vi "RelayControlPlottingSBE37andRTD.vi"() -> ()   [LabVIEW 2020]
uses:
  <vilib>/Utility/file.llb/Write Delimited Spreadsheet (string).vi
  <vilib>/Instr/_visa.llb/VISA Configure Serial Port (Instr).vi
  <vilib>/Utility/file.llb/Read Delimited Spreadsheet (string).vi
  75e3b035-2a18-8740-ad09-42cbc6dca646.vi
  3107c4ef-b790-5349-8479-afe5556ad064.vi
  <vilib>/picture/cartesn2.llb/XY Plot Type.ctl
panel:
  in  "setpoint":dbl format="%.2f"
  in  "XY plot cosmetics":T2={"plot color"=16776960, "XY plot type"=enum."connected points", "baseline"=0.0} {"baseline" format="%0.2f"}
  in  "cartesian axis attributes":T3={"x minimum"=0.0, "x maximum"=0.0, "x log?"=FALSE, "x precision"=1, "x format"=enum."Decimal", "y minimum"=0.0, "y maximum"=0.0, "y log?"=FALSE, "y precision"=1, "y format"=enum."Decimal"} {"x minimum" format="%0.2f"; "x maximum" format="%0.2f"; "y minimum" format="%0.2f"; "y maximum" format="%0.2f"}
  out "Table Control 2":string[][](table)
  out "2D Picture 3":picture
  out "Thermometer":dbl(slide) scale=0.0..100.0
  out "Table Control":string[][](table)
  out "2D Picture":picture
  out "Response":string
  out "?":u32
  in  "VISA resource name":refnum<visa-resource-name>="COM1"
  in  "error in (no error)":errorcluster
  in  "stop":bool
  in  "format (%s)":string="%s"
  out "error out":errorcluster
  in  "VISA resource name 2":refnum<visa-resource-name>
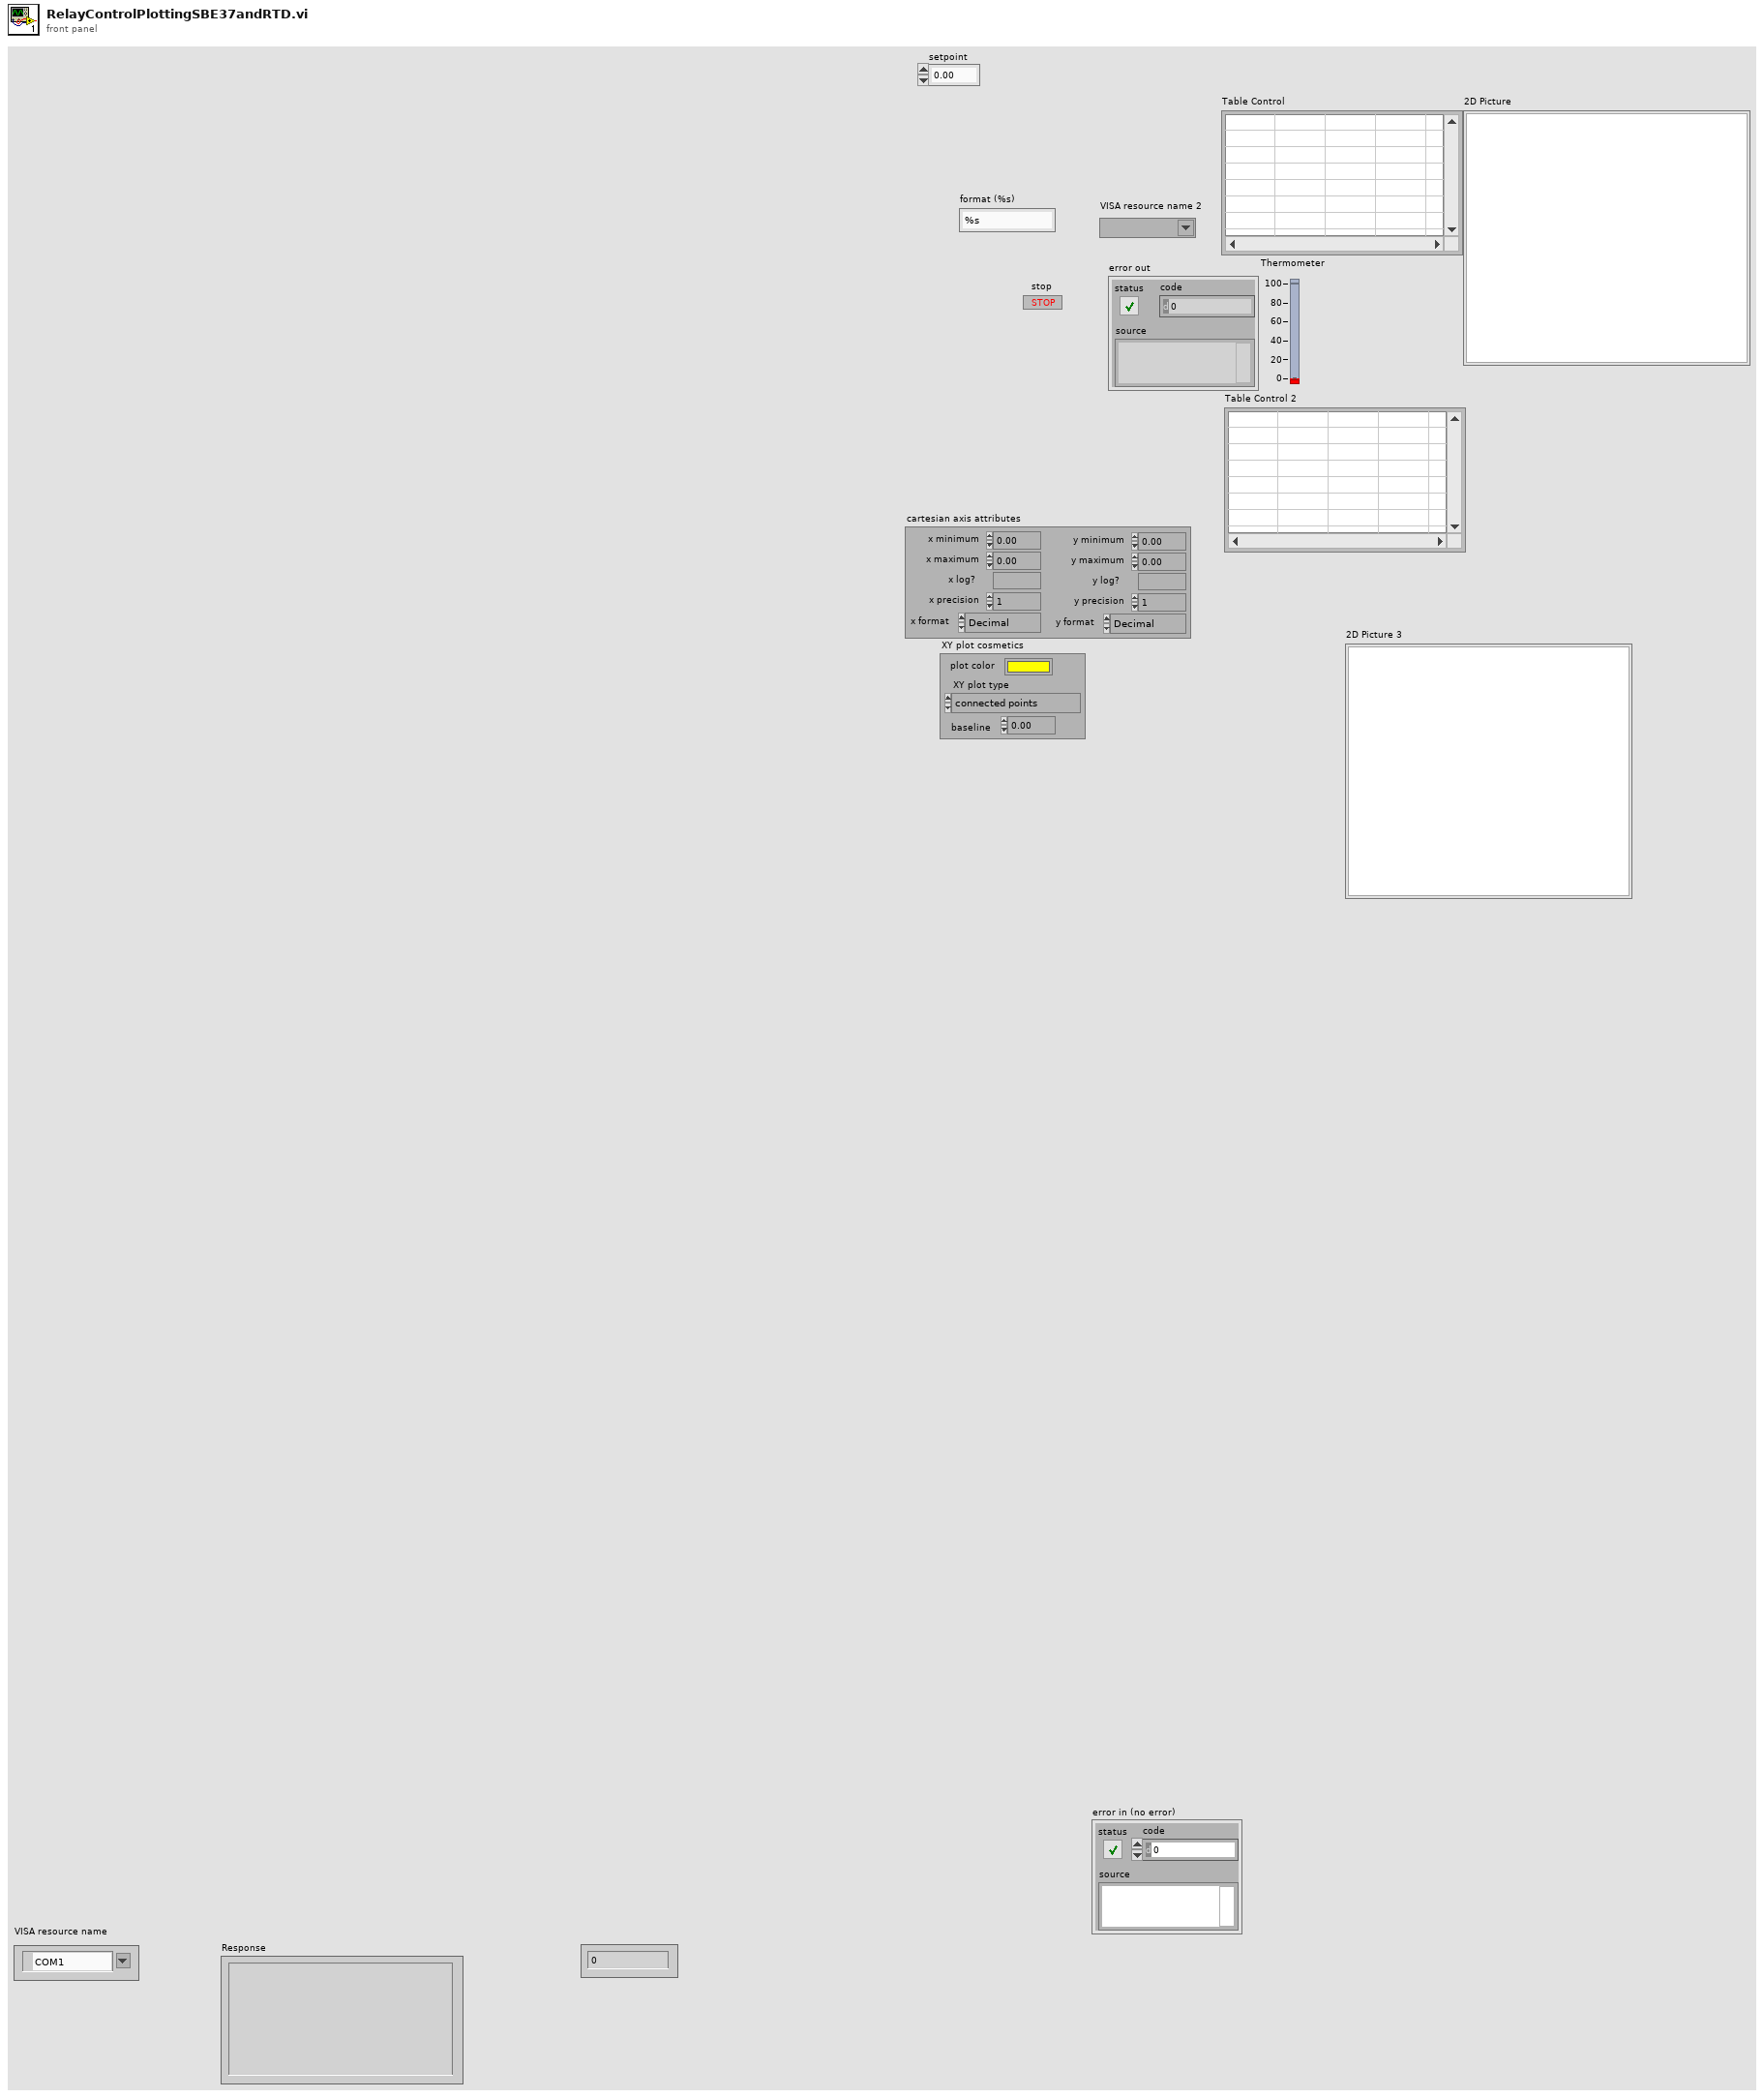
[diagram p1: front panel]
types:
  T1 = typedef "XY Plot Type.ctl" = enum16{"points", "squares", "circles", "connected points", "connected squares", "connected circles", "comb plot", "sized scatter plot", "sized-colored scatter plot", "min-max lines"}
  T2 = cluster{"plot color":u32, "XY plot type":T1, "baseline":dbl}
  T3 = cluster{"x minimum":dbl, "x maximum":dbl, "x log?":bool, "x precision":u8, "x format":enum8{"Decimal", "Scientific", "Engineering", "Binary", "Octal", "Hex"}, "y minimum":dbl, "y maximum":dbl, "y log?":bool, "y precision":u8, "y format":enum8{"Decimal", "Scientific", "Engineering", "Binary", "Octal", "Hex"}}
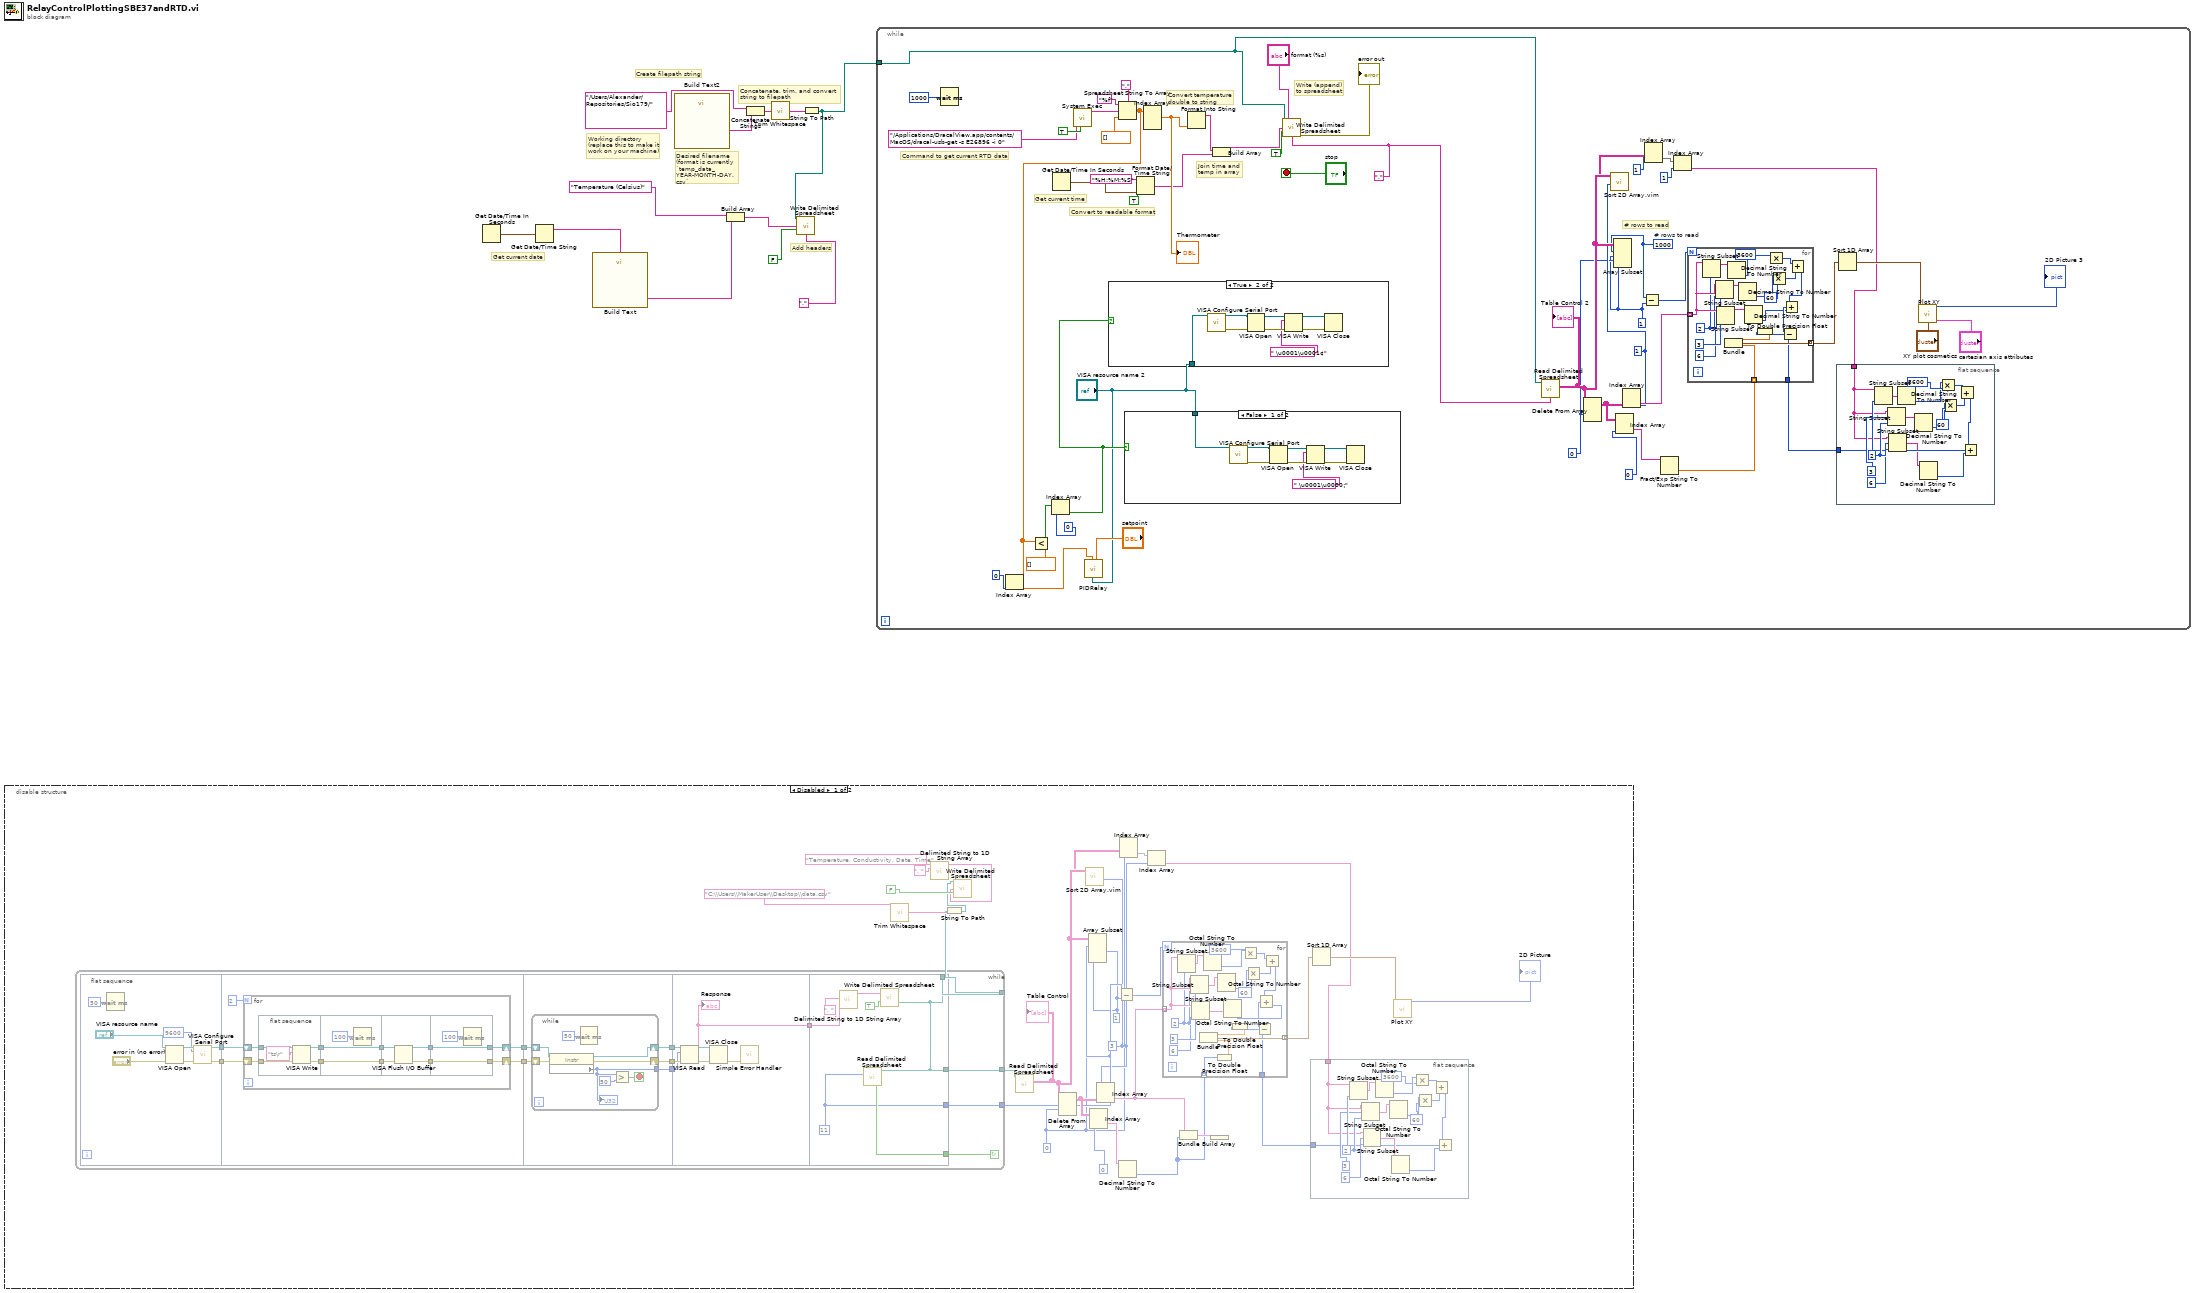
[diagram p0: block diagram]
diagram:
  # "Add headers"
  # "Get current date"
  # "Concatenate, trim, and convert string to filepath"
  # "Desired filename (format is currently `temp_data_YEAR-MONTH-DAY.csv`"
  # "Working directory (replace this to make it work on your machine)"
  # "Create filepath string"
  n1 = disable-structure shown="Disabled" {
    frame Disabled {
      w17 = 1
      w14 = 3
      w13 = 0
      n2 = call <vilib>:"Trim Whitespace.vi"("string"="C:\\Users\\MakerUser\\Desktop\\data.csv") -> ("trimmed string"=w38:string)  [unwired: 1 in]
      n3 = call <vilib>:"Delimited String to 1D String Array.vi"("delimiter"=", ", "delimited string"="Temperature, Conductivity, Date, Time") -> ("string array"=w35:string[])  [unwired: 9 in]
      n4 = String To Path(string=w38) -> (path=w32:path)
      n5 = while {
        tunnel: w32 -> [w81]
        tunnel: [w79] -> w31
        tunnel: [w78] -> w18
        stop <- w80 continue-if-true
        n6 = flat-sequence {
          tunnel: [w91] -> w89
          tunnel: [w90] -> w88
          tunnel: w89 -> [w102]
          tunnel: w88 -> [w101]
          tunnel: [w99] -> w87
          tunnel: [w98] -> w86
          tunnel: w87 -> [w132]
          tunnel: w86 -> [w131]
          tunnel: [w130] -> w85
          tunnel: [w129] -> w84
          tunnel: [w128] -> w83
          tunnel: w85 -> [w147]
          tunnel: w84 -> [w146]
          tunnel: w83 -> [w145]
          tunnel: [w141] -> w82
          tunnel: w82 -> [w154]
          tunnel: w81 -> [w149]
          tunnel: [w150] -> w80
          tunnel: [w149] -> w79
          tunnel: [w148] -> w78
          frame #0 {
            n7 = Wait (ms)(milliseconds to wait=50) -> ()  [unwired: 1 out]
            n8 = VISA Open(error in (no error)="error in (no error)", VISA resource name="VISA resource name") -> (VISA resource name=w95:refnum<visa-resource-name>, error out=w94:errorcluster)  [unwired: 3 in]
            n9 = call-poly "VISA Configure Serial Port"("VISA resource name"=w95, "baud rate (9600)"=u32 9600, "error in (no error)"=w94) -> ("VISA resource name out"=w91:refnum<visa-resource-name>, "error out"=w90:errorcluster)  [unwired: 6 in, 5 out]
          }
          frame #1 {
            n10 = for {
              N: 2 -> [_]
              shift-right: [w105] -> w99
              shift-left: w102 -> [w104]
              shift-right: [w106] -> w98
              shift-left: w101 -> [w103]
              n11 = flat-sequence {
                tunnel: w104 -> [w116]
                tunnel: w103 -> [w115]
                tunnel: [w114] -> w112
                tunnel: [w113] -> w109
                tunnel: w112 -> [w120]
                tunnel: [w120] -> w111
                tunnel: [w119] -> w110
                tunnel: w109 -> [w119]
                tunnel: w111 -> [w124]
                tunnel: w110 -> [w123]
                tunnel: [w122] -> w108
                tunnel: [w121] -> w107
                tunnel: [w127] -> w105
                tunnel: w108 -> [w127]
                tunnel: [w126] -> w106
                tunnel: w107 -> [w126]
                frame #0 {
                  n12 = VISA Write(VISA resource name=w116, write buffer="ts\r", error in (no error)=w115) -> (VISA resource name out=w113:refnum<visa-resource-name>, error out=w114:errorcluster)  [unwired: 1 out]
                }
                frame #1 {
                  n13 = Wait (ms)(milliseconds to wait=u32 100) -> ()  [unwired: 1 out]
                }
                frame #2 {
                  n14 = VISA Flush I/O Buffer(VISA resource name=w123, error in (no error)=w124) -> (VISA resource name out=w122:refnum<visa-resource-name>, error out=w121:errorcluster)  [unwired: 1 in]
                }
                frame #3 {
                  n15 = Wait (ms)(milliseconds to wait=u32 100) -> ()  [unwired: 1 out]
                }
              }
            }
          }
          frame #2 {
            n16 = while {
              tunnel: [w135] -> w128
              shift-right: [w138] -> w129
              shift-left: w131 -> [w133]
              shift-right: [w139] -> w130
              shift-left: w132 -> [w134]
              stop <- w136 stop-if-true
              n17 = property class="Instr"(reference=w134, error in=w133) -> (reference out=w139:refnum<visa-resource-name>, error out=w138:errorcluster, "Serial Settings:Number of Bytes at Serial Port"=w135:u32)
              "?" <- w135
              n18 = Wait (ms)(milliseconds to wait=50) -> ()  [unwired: 1 out]
              n19 = Greater?(x=w135, y=u32 50 ("Serial Settings:Number of Bytes at Serial Port")) -> (0:w136:bool)
            }
          }
          frame #3 {
            n20 = VISA Read(VISA resource name=w147, byte count=w145, error in (no error)=w146) -> (VISA resource name out=w143:refnum<visa-resource-name>, read buffer=w141:string, error out=w142:errorcluster)  [unwired: 1 out]
            "Response" <- w141
            n21 = VISA Close(VISA resource name=w143, error in (no error)=w142) -> (error out=w144:errorcluster)
            n22 = call <vilib>:"Simple Error Handler.vi"("error in (no error)"=w144) -> ()  [unwired: 1 in, 8 out]
          }
          frame #4 {
            w148 = 11
            n23 = call <vilib>:"Delimited String to 1D String Array.vi"("delimiter"=", ", "delimited string"=w154) -> ("string array"=w151:string[])  [unwired: 9 in]
            n24 = call-poly <vilib>:"Read Delimited Spreadsheet.vi"("file path (dialog if empty)"=w149, "number of rows (all:-1)"=w148) -> ("EOF?"=w150:bool)  [unwired: 8 in, 5 out]
            n25 = call-poly <vilib>:"Write Delimited Spreadsheet.vi"("file path (dialog if empty)"=w149, "1D data"=w151, "append to file? (new file:F)"=TRUE) -> ()  [unwired: 11 in, 2 out]
          }
        }
      }
      n26 = call-poly <vilib>:"Write Delimited Spreadsheet.vi"("file path (dialog if empty)"=w32, "1D data"=w35, "append to file? (new file:F)"=FALSE) -> ()  [unwired: 11 in, 2 out]
      n27 = call-poly <vilib>:"Read Delimited Spreadsheet.vi"("file path (dialog if empty)"=w31) -> ("all rows"=w16:string[][])  [unwired: 9 in, 5 out]
      "Table Control" <- w16
      n28 = Delete From Array(array=w16, index (row)=w13) -> (array with subset deleted=w30:string[][])  [unwired: 2 in, 1 out]
      n29 = call "Sort 2D Array.vim"("index"=w14, "2D array"=w16) -> ("sorted 2D array"=w15:string[][])  [unwired: 8 in, 1 out]
      n30 = Array Subset(array=w16, index (row)=w18, length (row)=w17, index (col)=w13, length (col)=w17) -> ()  [unwired: 1 out]
      n31 = Index Array(array=w30, index (col)=0) -> (element=w29:string[])  [unwired: 1 in]
      n32 = Index Array(array=w30, index (col)=w14) -> (element=w25:string[])  [unwired: 1 in]
      n33 = Subtract(x=w18, y=w17) -> (x-y=w27:i32)
      n34 = Decimal String To Number(string=w29) -> (number=w26:i32[])  [unwired: 2 in, 1 out]
      n35 = Index Array(array=w15, index (row)=w13) -> (element=w20:string[])  [unwired: 1 in]
      n36 = Index Array(array=w20, index=w14) -> (element=w19:string)
      n37 = for {
        N: w27 -> [_]
        tunnel: w26 -> [w76] mode=indexing
        tunnel: w25 -> [w73] mode=indexing
        tunnel: [w77] -> w23 mode=indexing
        tunnel: w21 -> [w56]
        w72 = 2
        n38 = String Subset(string=w73, length (rest)=w72) -> (substring=w67:string)  [unwired: 1 in]
        n39 = String Subset(string=w73, offset (0)=3, length (rest)=w72) -> (substring=w69:string)
        n40 = String Subset(string=w73, offset (0)=6, length (rest)=w72) -> (substring=w68:string)
        n41 = Octal String To Number(4:w67) -> (0:w66:u32)  [unwired: 2 in, 1 out]
        n42 = To Double Precision Float(number=w76) -> (double precision float=w75:dbl)
        n43 = Octal String To Number(4:w69) -> (0:w64:u32)  [unwired: 2 in, 1 out]
        n44 = Octal String To Number(4:w68) -> (0:w59:u32)  [unwired: 2 in, 1 out]
        n45 = Multiply(x=w66, y=3600) -> (x*y=w62:u32)
        n46 = Multiply(x=w64, y=60) -> (x*y=w61:u32)
        n47 = Add(x=w62, y=w61) -> (x+y=w60:u32)
        n48 = Add(x=w60, y=w59) -> (x+y=w58:u32)
        n49 = Subtract(x=w58, y=w56) -> (x-y=w57:u32)
        n50 = To Double Precision Float(number=w57) -> (double precision float=w74:dbl)
        n51 = Bundle(w74, w75) -> (w77:cluster{dbl, dbl})  [unwired: 1 in]
      }
      n52 = Bundle("all rows"=w25, w26) -> (w28:cluster{"all rows":string[], i32[]})  [unwired: 1 in]
      n53 = Build Array(w28) -> ()  [unwired: 1 out]
      n54 = flat-sequence {
        tunnel: [w41] -> w21
        tunnel: w19 -> [w40]
        frame #0 {
          w44 = 2
          n55 = String Subset(string=w40, length (rest)=w44) -> (substring=w53:string)  [unwired: 1 in]
          n56 = String Subset(string=w40, offset (0)=3, length (rest)=w44) -> (substring=w55:string)
          n57 = String Subset(string=w40, offset (0)=6, length (rest)=w44) -> (substring=w54:string)
          n58 = Octal String To Number(4:w53) -> (0:w52:u32)  [unwired: 2 in, 1 out]
          n59 = Octal String To Number(4:w55) -> (0:w51:u32)  [unwired: 2 in, 1 out]
          n60 = Octal String To Number(4:w54) -> (0:w48:u32)  [unwired: 2 in, 1 out]
          n61 = Multiply(x=w52, y=3600) -> (x*y=w50:u32)
          n62 = Multiply(x=w51, y=60) -> (x*y=w49:u32)
          n63 = Add(x=w50, y=w49) -> (x+y=w47:u32)
          n64 = Add(x=w47, y=w48) -> (x+y=w41:u32)
        }
      }
      n65 = Sort 1D Array(array=w23) -> (sorted array=w22:cluster{dbl, dbl}[])
      n66 = call <vilib>:"Plot XY.vi"("data"=w22) -> ("new picture"=→"2D Picture":picture)  [unwired: 14 in]
    }
    frame Enabled {
    }
  }
  n67 = Get Date/Time In Seconds() -> (seconds since 1Jan1904=w10:timestamp)
  n68 = Get Date/Time String(seconds (now)=w10) -> (date string=w6:string)  [unwired: 2 in, 1 out]
  n69 = call "Build Text"("date"=w6) -> ("Result"=w9:string)  [unwired: 13 in, 1 out]
  n70 = call "Build Text2"() -> ("Result"=w5:string)  [unwired: 14 in, 1 out]
  n71 = Build Array("Temperature (Celsius)", w9) -> (w8:string[])
  n72 = Concatenate Strings("/Users/Alexander/Repositories/Sio179/", w5) -> (w11:string)
  n73 = call <vilib>:"Trim Whitespace.vi"("string"=w11) -> ("trimmed string"=w12:string)  [unwired: 1 in]
  n74 = String To Path(string=w12) -> (path=w7:path)
  n75 = call-poly <vilib>:"Write Delimited Spreadsheet.vi"("file path (dialog if empty)"=w7, "1D data"=w8, "append to file? (new file:F)"=FALSE, "delimiter (\\t)"=",") -> ()  [unwired: 10 in, 2 out]
  n76 = while {
    tunnel: w7 -> [w174]
    stop <- "stop" stop-if-true
    w164 = ","
    w173 = 1000  # # rows to read
    w176 = 1
    w178 = 1
    w177 = 0
    # "# rows to read"
    # "Command to get current RTD data"
    # "Join time and temp in array"
    # "Convert temperature double to string"
    # "Convert to readable format"
    # "Get current time"
    # "Write (append) to spreadsheet"
    n77 = Wait (ms)(milliseconds to wait=u32 1000 ("millisecond timer value")) -> ()  [unwired: 1 out]
    n78 = Get Date/Time In Seconds() -> (seconds since 1Jan1904=w169:timestamp)
    n79 = call <vilib>:"System Exec.vi"("run minimized? (F)"=TRUE, "command line"="/Applications/DracalView.app/contents/MacOS/dracal-usb-get -s E26896 -i 0") -> ("standard output"=w201:string)  [unwired: 6 in, 3 out]
    n80 = Spreadsheet String To Array(delimiter (Tab)=",", format string="%f", spreadsheet string=w201, array type (2D Dbl)=dbl[] [] ("Array")) -> (array=w158:dbl[])
    n81 = Index Array(array=w158, index=0) -> (element=w157:dbl)
    n82 = Less?(x=w158, y=dbl[] []) -> (x < y?=w192:bool[])
    n83 = Index Array(array=w192, index=0) -> (element=w193:bool)
    n84 = call "PIDRelay.vi"("setpoint"="setpoint", "VISA resource name 2"="VISA resource name 2", "process variable"=w157) -> ()  [unwired: 9 in]
    n85 = case shown="True" w193 {
      tunnel: "VISA resource name 2" -> [_ w251]
      frame False {
      }
      frame True {
        n86 = call-poly "VISA Configure Serial Port"("VISA resource name"=w251) -> ("VISA resource name out"=w258:refnum<visa-resource-name>, "error out"=w257:errorcluster)  [unwired: 13 in]
        n87 = VISA Open(error in (no error)=w257, VISA resource name=w258) -> (VISA resource name=w256:refnum<visa-resource-name>, error out=w255:errorcluster)  [unwired: 3 in]
        n88 = VISA Write(VISA resource name=w256, write buffer=" \u0001\u0001¢", error in (no error)=w255) -> (VISA resource name out=w254:refnum<visa-resource-name>, error out=w253:errorcluster)  [unwired: 1 out]
        n89 = VISA Close(VISA resource name=w254, error in (no error)=w253) -> ()  [unwired: 1 out]
      }
    }
    n90 = case shown="False" w193 {
      tunnel: "VISA resource name 2" -> [w243 _]
      frame False {
        n91 = call-poly "VISA Configure Serial Port"("VISA resource name"=w243) -> ("VISA resource name out"=w250:refnum<visa-resource-name>, "error out"=w249:errorcluster)  [unwired: 13 in]
        n92 = VISA Open(error in (no error)=w249, VISA resource name=w250) -> (VISA resource name=w248:refnum<visa-resource-name>, error out=w247:errorcluster)  [unwired: 3 in]
        n93 = VISA Write(VISA resource name=w248, write buffer=" \u0001\u0000¡", error in (no error)=w247) -> (VISA resource name out=w246:refnum<visa-resource-name>, error out=w245:errorcluster)  [unwired: 1 out]
        n94 = VISA Close(VISA resource name=w246, error in (no error)=w245) -> ()  [unwired: 1 out]
      }
      frame True {
      }
    }
    n95 = Format Date/Time String(time format string (%c)="%H:%M:%S", seconds (now)=w169, UTC format=TRUE) -> (date/time string=w172:string)
    n96 = Index Array(array=w158) -> (element #1=w190:dbl)  [unwired: 3 in, 2 out]
    "Thermometer" <- w190
    n97 = Format Into String(w190) -> (resulting string=w194:string)  [unwired: 3 in, 1 out]
    n98 = Build Array(w194, w172) -> (w195:string[])
    n99 = call-poly <vilib>:"Write Delimited Spreadsheet.vi"("file path (dialog if empty)"=w174, "format (%s)"="format (%s)", "1D data"=w195, "append to file? (new file:F)"=TRUE, "delimiter (\\t)"=w164) -> ("error out"=→"error out":errorcluster)  [unwired: 9 in, 1 out]
    n100 = call-poly <vilib>:"Read Delimited Spreadsheet.vi"("file path (dialog if empty)"=w174, "delimiter (\\t)"=w164) -> ("all rows"=w180:string[][])  [unwired: 8 in, 5 out]
    "Table Control 2" <- w180
    n101 = Delete From Array(array=w180, index (row)=w177) -> (array with subset deleted=w189:string[][])  [unwired: 2 in, 1 out]
    n102 = call "Sort 2D Array.vim"("index"=w178, "2D array"=w180) -> ("sorted 2D array"=w179:string[][])  [unwired: 8 in, 1 out]
    n103 = Array Subset(array=w180, index (row)=w173, length (row)=w176, index (col)=w177, length (col)=w176) -> ()  [unwired: 1 out]
    n104 = Index Array(array=w189, index (col)=0) -> (element=w168:string[])  [unwired: 1 in]
    n105 = Index Array(array=w189, index (col)=w178) -> (element=w187:string[])  [unwired: 1 in]
    n106 = Subtract(x=w173, y=w176) -> (x-y=w188:i32)
    n107 = Index Array(array=w179, index (row)=1) -> (element=w182:string[])  [unwired: 1 in]
    n108 = Fract/Exp String To Number(string=w168) -> (number=w167:dbl[])  [unwired: 3 in, 1 out]
    n109 = Index Array(array=w182, index=1) -> (element=w181:string)
    n110 = for {
      N: w188 -> [_]
      tunnel: w187 -> [w240] mode=indexing
      tunnel: [w242] -> w185 mode=indexing
      tunnel: w183 -> [w229]
      tunnel: w167 -> [w222] mode=indexing
      w239 = 2
      n111 = String Subset(string=w240, length (rest)=w239) -> (substring=w223:string)  [unwired: 1 in]
      n112 = String Subset(string=w240, offset (0)=3, length (rest)=w239) -> (substring=w226:string)
      n113 = String Subset(string=w240, offset (0)=6, length (rest)=w239) -> (substring=w227:string)
      n114 = Decimal String To Number(string=w223) -> (number=w224:i32)  [unwired: 2 in, 1 out]
      n115 = Decimal String To Number(string=w226) -> (number=w225:i32)  [unwired: 2 in, 1 out]
      n116 = Decimal String To Number(string=w227) -> (number=w228:i32)  [unwired: 2 in, 1 out]
      n117 = Multiply(x=w224, y=3600) -> (x*y=w234:i32)
      n118 = Multiply(x=w225, y=60) -> (x*y=w233:i32)
      n119 = Add(x=w234, y=w233) -> (x+y=w232:i32)
      n120 = Add(x=w232, y=w228) -> (x+y=w231:i32)
      n121 = Subtract(x=w231, y=w229) -> (x-y=w230:i32)
      n122 = To Double Precision Float(number=w230) -> (double precision float=w241:dbl)
      n123 = Bundle(w241, "String"=w222) -> (w242:cluster{dbl, "String":dbl})  [unwired: 1 in]
    }
    n124 = flat-sequence {
      tunnel: [w213] -> w183
      tunnel: w181 -> [w212]
      frame #0 {
        w216 = 2
        n125 = String Subset(string=w212, length (rest)=w216) -> (substring=w209:string)  [unwired: 1 in]
        n126 = String Subset(string=w212, offset (0)=3, length (rest)=w216) -> (substring=w210:string)
        n127 = String Subset(string=w212, offset (0)=6, length (rest)=w216) -> (substring=w211:string)
        n128 = Decimal String To Number(string=w209) -> (number=w208:i32)  [unwired: 2 in, 1 out]
        n129 = Decimal String To Number(string=w210) -> (number=w207:i32)  [unwired: 2 in, 1 out]
        n130 = Decimal String To Number(string=w211) -> (number=w206:i32)  [unwired: 2 in, 1 out]
        n131 = Multiply(x=w208, y=3600) -> (x*y=w221:i32)
        n132 = Multiply(x=w207, y=60) -> (x*y=w220:i32)
        n133 = Add(x=w221, y=w220) -> (x+y=w219:i32)
        n134 = Add(x=w219, y=w206) -> (x+y=w213:i32)
      }
    }
    n135 = Sort 1D Array(array=w185) -> (sorted array=w184:cluster{dbl, "String":dbl}[])
    n136 = call <vilib>:"Plot XY.vi"("data"=w184, "cartesian axis attributes"="cartesian axis attributes", "XY plot cosmetics"="XY plot cosmetics") -> ("new picture"=→"2D Picture 3":picture)  [unwired: 12 in]
  }
